vi "Dashboard Main.vi"() -> ()   [LabVIEW 2015]
uses:
  <vilib>/Utility/miscctls.llb/LVRowAndColumnTypeDef.ctl
  <vilib>/event_ctls.llb/eventvkey.ctl
  <vilib>/Rock Robotics/WPI/Dashboard/WPI_DashboardLogging Global.vi
  <vilib>/Rock Robotics/Network Tables/NT Read Numeric Array.vi
  <vilib>/Utility/config.llb/Write Key (String).vi
  <vilib>/Utility/config.llb/Write Key (I32).vi
  <vilib>/Utility/config.llb/NI_LVConfig.lvlib
panel:
  in  "TCP":refnum<k5>
  in  "Rec Mode":enum32{"Stop", "Record", "Playback"}(radio)
  in  "Vision":u16(ring) items=["Camera Off", "USB Camera SW", "USB Camera HW", "IP Camera"]
  out "Camera IP":string
  out "Image Message":string="Timeout in Camera Communications"
  in  "Dashboard Tab":T1(tab)
  in  "Select Auto":string(combo)
  out "NT Connection":bool
  in  "Camera Settings":T2={"Frame Rate"=30, "Compression"=30, "Size"=1} {"Frame Rate" scale=1.0..30.0; "Size" items=["640x480", "320x240", "160x120"]}
  out "MotorChart R":cluster{"Numeric":dbl, "Numeric":dbl}(graph)
  out "MotorChart L":T3(graph)
  out "MotorSliders R":cluster{"MotorSlide1":dbl, "MotorSlide2":dbl} {"MotorSlide2" scale=-1.0..1.0 scale format="%#_2e"; "MotorSlide1" scale=-1.0..1.0 scale format="%#_2e"}
  out "MotorSliders L":T4 {"MotorSlide4 2" scale=0.0..14.0 scale format="%#_2e"; "MotorSlide2" scale=-1.0..1.0 scale format="%#_2e"; "MotorSlide1" scale=-1.0..1.0 scale format="%#_2e"}
  out "Gyro":dbl(knob) scale=0.0..360.0
  out "JS1 Z":dbl(slide) scale=-1.0..1.0 scale format="%#_2e"
  out "JS1 Graph":cluster{"X":dbl, "Y":dbl}[](graph)
  out "JS1 Buttons":T5
  out "JS2 Z":dbl(slide) scale=-1.0..1.0 scale format="%#_2e"
  out "JS2 Graph":cluster{"X":dbl, "Y":dbl}[](graph)
  out "JS2 Buttons":T5
  out "Mode":T6(ring)=enum."Auto Disabled"
  in  "DB Camera Config":bool
  out "fps":dbl format="%#.1g"
  out "Mbps":dbl format="%#.1g"
  out "Mbps LED":bool
  in  "Auto-Mode":T7(ring)
  out "Satellite Speed":dbl(knob) scale=0.0..1.0
  out "Uranus Rotation in Degrees":dbl(knob) scale=0.0..360.0
  out "Uranus Distance":dbl
  out "Uranus Direction":bool
  out "Uranus Rate":dbl
  in  "Test Slider":dbl(slide) scale=0.0..100.0 scale format="%#_3g"
  in  "On/Off":bool caption="Solenoid"
  in  "Test Name":u16(ring) items=["Select the test to run..."]
  in  "Test Tree":string(tree)
  in  "Motor":cluster{"Value":dbl, "Enable":bool} {"Value" scale=-1.0..1.0 scale format="%#_3g"}
  out "Progress":T8 {"Test Progress" scale=0.0..100.0}
  in  "Rev/Fwd":cluster{"Forward":bool, "Reverse":bool}
  in  "Test Ring":u16(ring) items=["Monochrome", "Color"]
  out "Cmd Status":string
  in  "Execute Command":bool
  in  "Command Params":string[][](table)
  in  "Command Selection":i32(listbox)
  in  "CheckList":i32(listbox)
  out "Tree":string(tree)
  out "Camera Image":T9(plugin-control)
  out "Background":bool
  # "Left"
  # "Front"
  # "Right"
  # "Battery"
  # "This tab is a great place for autonomous settings and robot-specific values.\nPlace controls and indicators inside this tab and match name to\nDashboard Variables on robot. You can also delete this comment."
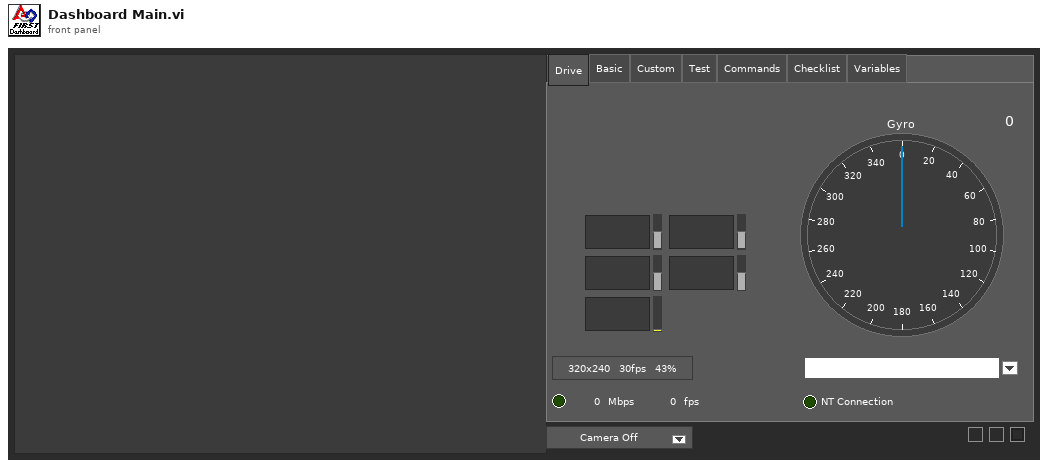
[diagram p1: front panel]
types:
  T1 = enum32{"Drive", "Basic", "Custom", "Test", "Commands", "Checklist", "Variables"}
  T2 = cluster{"Frame Rate":i32, "Compression":i32, "Size":u16}
  T3 = cluster{"Numeric":dbl, "Numeric":dbl, "Battery V":dbl}
  T4 = cluster{"MotorSlide1":dbl, "MotorSlide2":dbl, "MotorSlide4 2":dbl}
  T5 = cluster{bool, bool, bool, bool, bool, bool, bool, bool, bool, bool, bool, bool}
  T6 = enum8{"Tele-Op Disabled", "Tele-Op Enabled", "Auto Disabled", "Auto Enabled", "Test Disabled", "Test Enabled", "Disconnected", "No Code", "E-Stop"}
  T7 = enum16{"Drive-Over Stuff", "Drawbridge", "Portiwhatnot"}
  T8 = cluster{"Test Progress":u8, "Test Progress Text":string}
  T9 = typedef "IMAQ Image.ctl" = refnum<image>
  T10 = cluster{"IDs":cluster{"RPC field ID":u16, "Unique ID":u16}, "String":string}
  T11 = enum32{"Drive", "Basic", "Custom", "Test", "Checklist", "Variables"}
  T12 = typedef "Image Type" = u32
  T13 = cluster{"Camera Image":refnum<vi>, "Dashboard Tab":refnum<vi>, "Background":refnum<vi>, "Vision":refnum<vi>, "Rec Mode":refnum<vi>, "Test Slider":refnum<vi>, "On/Off ":refnum<vi>, "Test Ring":refnum<vi>, "Rev/Fwd":refnum<vi>, "Test Name":refnum<vi>, "Motor":refnum<vi>, "Progress":refnum<vi>, "CheckList":refnum<vi>, "Tree":refnum<vi>, "Test Tree":refnum<vi>, "Command Params":refnum<vi>, "Command Selection":refnum<vi>, "Execute Command":refnum<vi>, "Cmd Status":refnum<vi>}
  T14 = cluster{"Error Strings":string, "Disable Counts":cluster{u16, u16}, "Rail Faults":cluster{u16, u16, u16}, "Robot IP":string, "DB Mode":u8, "Event Info":cluster{"Name":string, "Type":u8, "Number":u16, "Replay":u8}, "Camera Addr":string}
  T15 = cluster{"Storage":cluster{"Disk Free":u64, "RAM Block":u32, "RAM free":u32}, "CPU Utilization":cluster{"CPU % ISR":sgl, "CPU % Time Crit":sgl, "CPU % Timed Str":sgl, "CPU % High":sgl, "CPU % Above":sgl, "CPU % Normal":sgl, "CPU % Low":sgl}, "CAN":cluster{"% Bus Utilization":sgl, "Bus Off Cnt":u32, "TX_FIFO Full Cnt":u32, "Receive Error Cnt":u8, "Transmit Error Cnt":u8}, "HID":cluster{"HID Outputs":u32, "Rumble Low":u16, "Rumble High":u16}[]}
  T16 = cluster{"Status bits":cluster{"Test Mode":bool, "Autonomous":bool, "Enabled":bool, "Code Start":bool, "Brownout":bool, "Reserved 2":bool, "Reserved 3":bool, "E-Stop":bool}, "Code Trace":cluster{"Disabled":bool, "TeleOp":bool, "Auto":bool, "Test":bool}, "Controller Type":enum16{"unknown", "cRIO", "roboRio"}, "Code?":enum16{"unknown", "noCode", "code"}, "Battery V":dbl}
  T17 = cluster{"Control Bits":cluster{"TestMode":bool, "Autonomous":bool, "Enabled":bool, "FMS Present":bool, bool, bool, bool, "E-Stop":bool}, "Team Station ":u8, "Countdown":sgl, "Joystick Values":cluster{"Axes":dbl[], "Buttons":bool[], "POVs":i16[]}[]}
  T18 = cluster{"Axes":dbl[], "Buttons":bool[], "POVs":i16[]}[]
  T19 = cluster{"Axes":dbl[], "Buttons":bool[], "POVs":i16[]}
  T20 = cluster{"Buttons[0]":bool, "Buttons[1]":bool, "Buttons[2]":bool, "Buttons[3]":bool, "Buttons[4]":bool, "Buttons[5]":bool, "Buttons[6]":bool, "Buttons[7]":bool, "Buttons[8]":bool, "Buttons[9]":bool, "Buttons[10]":bool, "Buttons[11]":bool}
  T21 = typedef "NI_LVConfig.lvlib/Config Data RefNum.ctl" = refnum<k1>
  T22 = cluster{"Operation":enum16{"Update", "Clear"}, "Color Box":u32}[]
  T23 = typedef "eventvkey.ctl" = enum16{"ASCII", "Enter", "Return", "Shift", "Ctrl", "Alt", "Cmd", "Opt", "Caps", "NumLock", "Clear", "Break", "Up", "Down", "Left", "Right", "Insert", "Delete", "Home", "End", "PageUp", "PageDown", "Escape", "Help", "Pause", "ScrollLock", "F1", "F2", "F3", "F4", "F5", "F6", "F7", "F8", "F9", "F10", "F11", "F12", "F13", "F14", "F15", "F16", "F17", "F18", "F19", "F20", "F21", "F22", "F23", "F24", "Play", "VolumeUp", "VolumeDown", "Mute", "Two Byte Char"}
  T24 = cluster{"Image Size":bool, "Image Type":bool, "Pixel Value":bool, "ROI Information":bool, "Zoom Factor":bool}
  T25 = enum8{"Enabled", "Disabled", "Disabled and Grayed Out"}
  T26 = cluster{"Operation":enum16{"Update", "Clear"}, "Color Box":u32}
  T27 = typedef "LVRowAndColumnTypeDef.ctl" = cluster{"Row":i32, "Column":i32}
  T28 = cluster{"Shift":bool, "Ctrl":bool, "Alt":bool, "Cmd":bool, "Opt":bool}
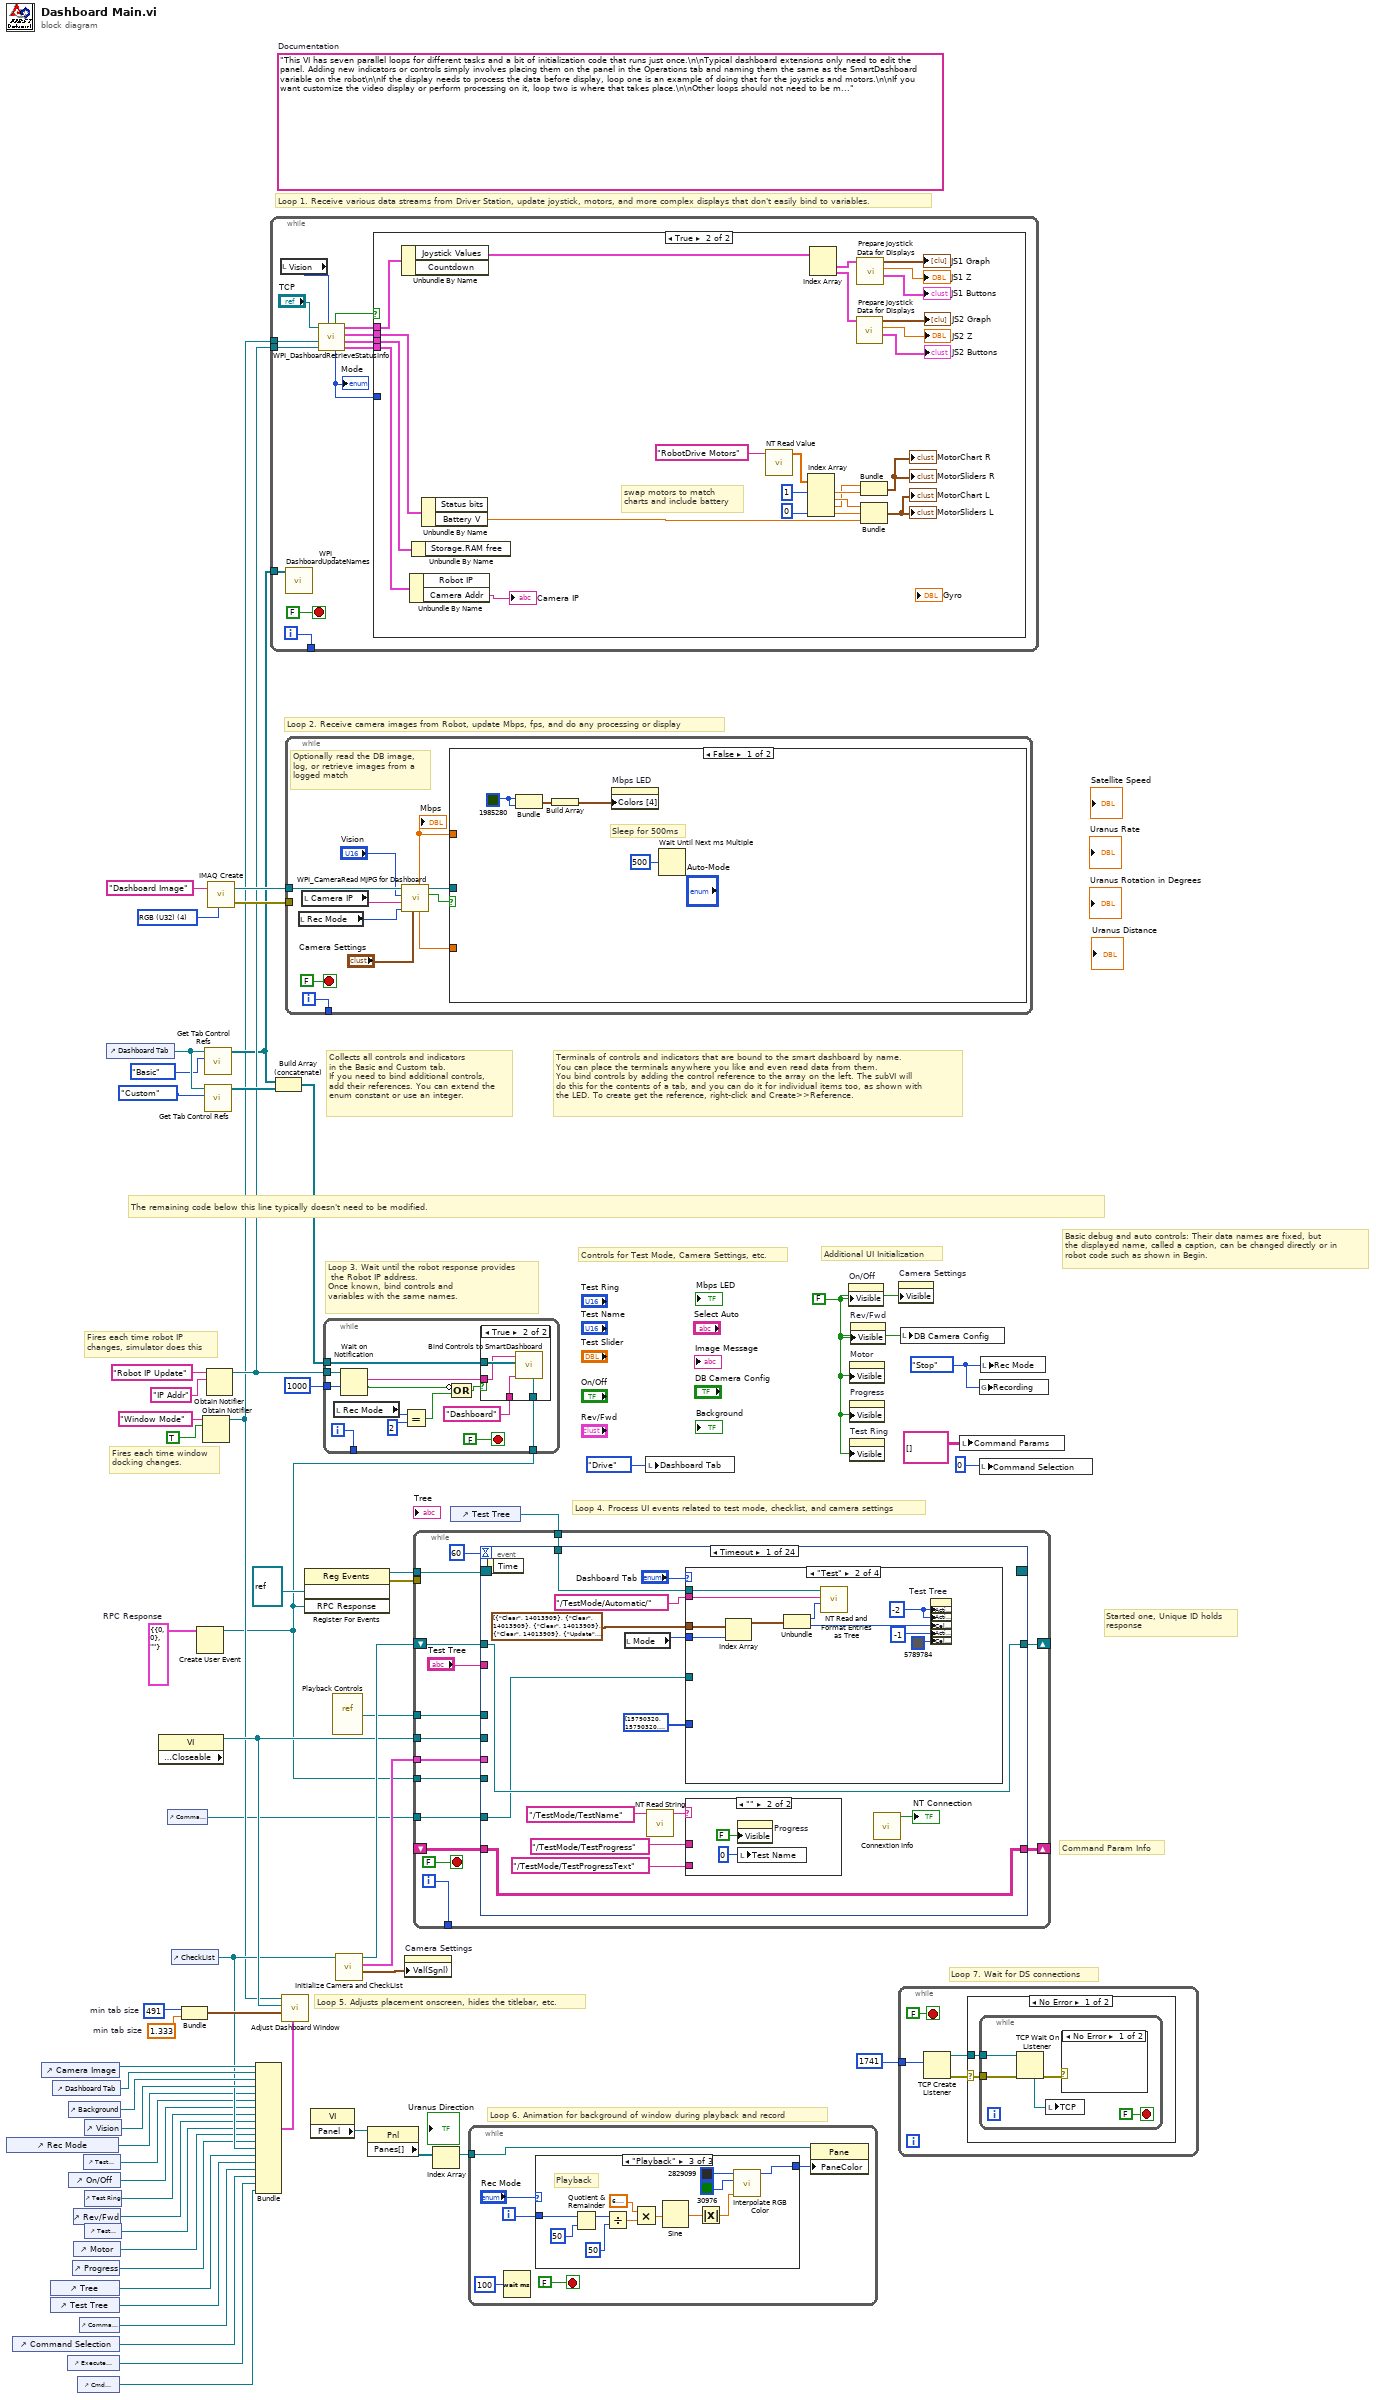
[diagram p0: block diagram]
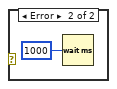
[diagram p2: hidden frame]
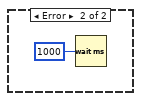
[diagram p3: hidden frame]
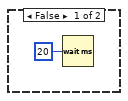
[diagram p4: hidden frame]
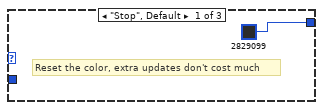
[diagram p5: hidden frame]
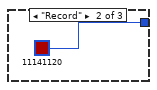
[diagram p6: hidden frame]
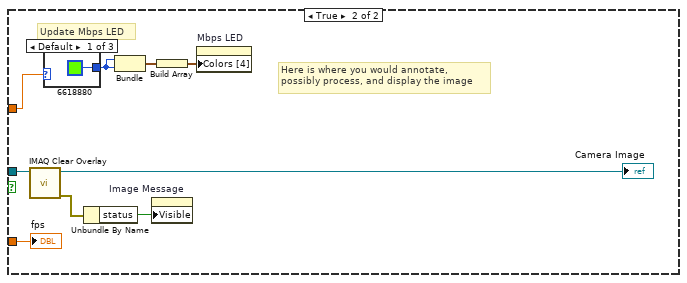
[diagram p8: hidden frame]
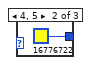
[diagram p9: hidden frame]
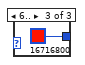
[diagram p10: hidden frame]
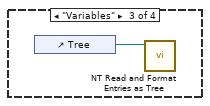
[diagram p12: hidden frame]
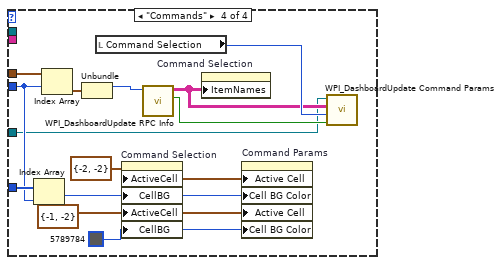
[diagram p13: hidden frame]
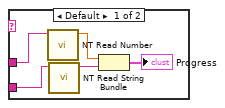
[diagram p14: hidden frame]
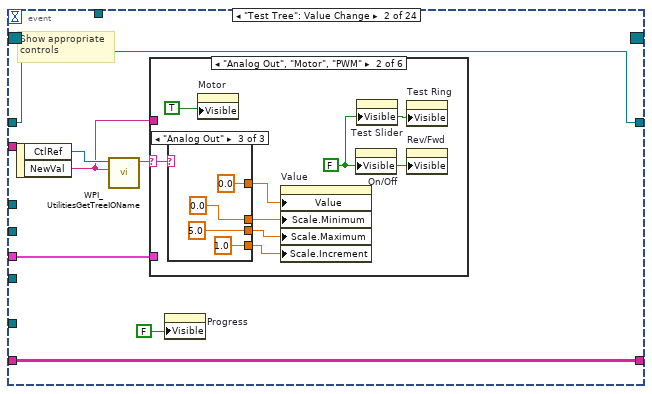
[diagram p15: hidden frame]
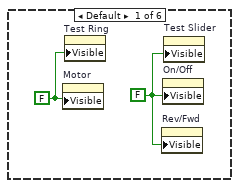
[diagram p16: hidden frame]
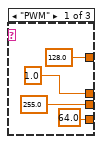
[diagram p17: hidden frame]
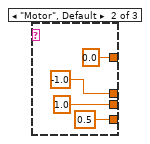
[diagram p18: hidden frame]
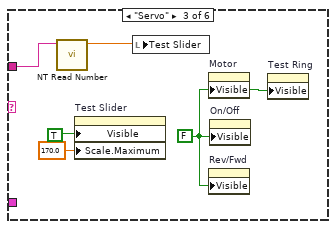
[diagram p19: hidden frame]
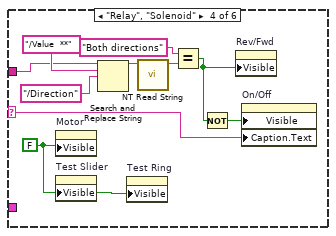
[diagram p20: hidden frame]
diagram:
  w7 = T10 {"IDs"={"RPC field ID"=0, "Unique ID"=0}, "String"=""}  # RPC Response
  w33 = 491  # min tab size
  w32 = 1.333  # min tab size
  w41 = enum32{"Stop", "Record", "Playback"}."Stop" ("Rec Mode")
  w15 = FALSE ("Visible")
  (unwired) "This VI has seven parallel loops for different tasks and a bit of initialization code that runs just once.\n\nTypical dashboard extensions only need to edit the panel. Adding new indicators or controls simply involves placing them on the panel in the Operations tab and naming them the same as the SmartDashboard variable on the robot\n\nIf the display needs to process the data before display, loop one is an example of doing that for the joysticks and motors.\n\nIf you want customize the video display or perform processing on it, loop two is where that takes place.\n\nOther loops should not need to be modified. They are pretty standard, and document the task they perform."  # Documentation
  w61 = T12 4 items=["Grayscale (U8)", "Grayscale (I16)", "Grayscale (SGL)", "Complex (CSG)", "RGB (U32)", "HSL (U32)", "RGB (U64)"] ("Image Type")
  # "Command Param Info"
  # "Started one, Unique ID holds\nresponse"
  # "Loop 7. Wait for DS connections"
  # "Basic debug and auto controls: Their data names are fixed, but\nthe displayed name, called a caption, can be changed directly or in\nrobot code such as shown in Begin."
  # "Controls for Test Mode, Camera Settings, etc."
  # "Additional UI Initialization"
  # "Loop 6. Animation for background of window during playback and record"
  # "Fires each time robot IP\nchanges, simulator does this"
  # "Fires each time window\ndocking changes."
  # "Collects all controls and indicators\nin the Basic and Custom tab.\nIf you need to bind additional controls,\nadd their references. You can extend the\nenum constant or use an integer."
  # "The remaining code below this line typically doesn't need to be modified."
  # "Loop 4. Process UI events related to test mode, checklist, and camera settings"
  # "Terminals of controls and indicators that are bound to the smart dashboard by name.\nYou can place the terminals anywhere you like and even read data from them.\nYou bind controls by adding the control reference to the array on the left. The subVI will\ndo this for the contents of a tab, and you can do it for individual items too, as shown with\nthe LED. To create get the reference, right-click and Create>>Reference."
  # "Loop 3. Wait until the robot response provides\n the Robot IP address.\nOnce known, bind controls and\nvariables with the same names."
  # "Loop 5. Adjusts placement onscreen, hides the titlebar, etc."
  # "Loop 1. Receive various data streams from Driver Station, update joystick, motors, and more complex displays that don't easily bind to variables."
  # "Loop 2. Receive camera images from Robot, update Mbps, fps, and do any processing or display"
  n1 = control-ref of="Rec Mode"() -> (w21:refnum<vi>)
  n2 = control-ref of="Command Selection"() -> (w6:refnum<vi>)
  n3 = control-ref of="Camera Image"() -> (w36:refnum<vi>)
  n4 = control-ref of="Tree"() -> (w25:refnum<vi>)
  n5 = control-ref of="Test Tree"() -> (w24:refnum<vi>)
  n6 = control-ref of="Dashboard Tab"() -> (w35:refnum<vi>)
  n7 = control-ref of="Execute Command"() -> (w8:refnum<vi>)
  n8 = control-ref of="Background"() -> (w30:refnum<vi>)
  n9 = control-ref of="On/Off"() -> (w19:refnum<vi>)
  n10 = control-ref of="Progress"() -> (w16:refnum<vi>)
  n11 = control-ref of="Rev/Fwd"() -> (w17:refnum<vi>)
  n12 = control-ref of="Motor"() -> (w22:refnum<vi>)
  n13 = control-ref of="Cmd Status"() -> (w2:refnum<vi>)
  n14 = control-ref of="Command Params"() -> (w9:refnum<vi>)
  n15 = control-ref of="Test Slider"() -> (w20:refnum<vi>)
  n16 = control-ref of="Vision"() -> (w34:refnum<vi>)
  n17 = control-ref of="Test Ring"() -> (w18:refnum<vi>)
  n18 = control-ref of="Test Name"() -> (w23:refnum<vi>)
  n19 = control-ref of="Dashboard Tab"() -> (w39:refnum<vi>)
  n20 = property class="VI" props=["Front Panel.Closeable"]() -> (reference out=w40:refnum<vi>)  [unwired: 2 in, 2 out]
  n21 = control-ref of="Command Params"() -> (w1:refnum<vi>)
  n22 = control-ref of="CheckList"() -> (w26:refnum<vi>)
  n23 = Bundle("min tab size"=w33, "min tab size"=w32) -> (w31:cluster{"min tab size":i32, "min tab size":dbl})  [unwired: 1 in]
  n24 = Create User Event(user event datatype=w7) -> (user event=w3:refnum<user-event>)  [unwired: 1 in, 1 out]
  n25 = Obtain Notifier(name (unnamed)="Window Mode", notification data type=TRUE) -> (notifier out=w12:refnum<notifier>)  [unwired: 2 in, 2 out]
  n26 = call <vilib>:"Get Tab Control Refs.vi"("Page Index"=T11."Basic" ("Dashboard Tab"), "TabControl in"=w39) -> ("ControlsOnPage"=w13:refnum<vi>[])  [unwired: 9 in]
  n27 = call <vilib>:"Get Tab Control Refs.vi"("Page Index"=T11."Custom" ("Dashboard Tab"), "TabControl in"=w39) -> ("ControlsOnPage"=w38:refnum<vi>[])  [unwired: 9 in]
  n28 = Obtain Notifier(name (unnamed)="Robot IP Update", notification data type="IP Addr" ("name (unnamed)")) -> (notifier out=w14:refnum<notifier>)  [unwired: 2 in, 2 out]
  n29 = call "IMAQ Create"("Image Name"="Dashboard Image", "Image Type"=w61) -> ("New Image"=w59:T9, "error out"=w58:errorcluster)  [unwired: 2 in, 1 out]
  n30 = Bundle("Camera Image"=w36, "Dashboard Tab"=w35, "Background"=w30, "Vision"=w34, "Rec Mode"=w21, "Test Slider"=w20, "On/Off"=w19, "Test Ring"=w18, "Rev/Fwd"=w17, "Test Name"=w23, "Motor"=w22, "Progress"=w16, "CheckList"=w26, "Tree"=w25, "Test Tree"=w24, "Command Params"=w9, "Command Selection"=w6, "Execute Command"=w8, "Cmd Status"=w2) -> (w27:T13)  [unwired: 1 in]
  n31 = while {
    tunnel: [w73] -> _
    tunnel: w14 -> [w67]
    tunnel: w13 -> [w66]
    tunnel: w12 -> [w62]
    i -> [w73]
    stop <- FALSE stop-if-true
    n32 = local read "Vision"() -> (w64:u16)
    n33 = call <vilib>:"WPI_DashboardUpdateNames.vi"("Controls on Tab"=w66) -> ()  [unwired: 11 in]
    n34 = call <vilib>:"WPI_DashboardRetrieveStatusInfo.vi"("Vision"=w64, "Binding Refnum"=w67, "Window Mode Notifier"=w62, "TCP Cnx"="TCP") -> ("Power and Errors"=w68:T14, "Robot Metrics"=w71:T15, "Status Info"=w72:T16, "Control Info"=w69:T17, "Robot Mode"=w65:T6, "Process?"=w70:bool)  [unwired: 2 in]
    "Mode" <- w65
    n35 = case shown="True" w70 {
      tunnel: w72 -> [_ w100]
      tunnel: w71 -> [_ w99]
      tunnel: w69 -> [_ w98]
      tunnel: w68 -> [_ w97]
      tunnel: w65 -> [_ _]
      frame False {
        n36 = Wait (ms)(milliseconds to wait=u32 20) -> ()  [unwired: 1 out]
      }
      frame True {
        # "swap motors to match\ncharts and include battery"
        n37 = Unbundle By Name(w98) -> ("Joystick Values"=w87:T18)  [unwired: 1 out]
        n38 = Unbundle By Name(w97) -> ("Camera Addr"=→"Camera IP":string)  [unwired: 1 out]
        n39 = Unbundle By Name(w99) -> ()  [unwired: 1 out]
        n40 = Unbundle By Name(w100) -> ("Battery V"=w88:dbl)  [unwired: 1 out]
        n41 = call-poly <vilib>:"NT Read Value.vi"("Name"="RobotDrive Motors") -> ("Numeric Array"=w76:dbl[])  [unwired: 9 in, 1 out]
        n42 = Index Array(array=w76, index #1=1, index #4=0) -> (element #1=w92:dbl, element #2=w93:dbl, element #3=w91:dbl, element #4=w96:dbl)  [unwired: 2 in]
        n43 = Index Array(array=w87) -> (element #1=w86:T19, element #2=w81:T19)  [unwired: 2 in]
        n44 = call "Prepare Joystick Data for Displays.vi"("Joystick Values"=w81) -> ("Buttons"=→"JS2 Buttons":T20, "Z Axis"=→"JS2 Z":dbl, "Cartesian Data"=→"JS2 Graph":cluster{"X axis":dbl, "X axis":dbl}[])  [unwired: 8 in]
        n45 = call "Prepare Joystick Data for Displays.vi"("Joystick Values"=w86) -> ("Buttons"=→"JS1 Buttons":T20, "Z Axis"=→"JS1 Z":dbl, "Cartesian Data"=→"JS1 Graph":cluster{"X axis":dbl, "X axis":dbl}[])  [unwired: 8 in]
        n46 = Bundle("Numeric"=w91, "Numeric"=w92) -> (→"MotorChart R" →"MotorSliders R":cluster{"Numeric":dbl, "Numeric":dbl})  [unwired: 1 in]
        n47 = Bundle("Numeric"=w93, "Numeric"=w96, "Battery V"=w88) -> (→"MotorChart L" →"MotorSliders L":T3)  [unwired: 1 in]
      }
    }
  }
  n48 = Build Array (concatenate)(w13, w38) -> (w37:refnum<vi>[])
  n49 = call "Adjust Dashboard Window.vi"("Sizing Refnums"=w27, "Size Constraints"=w31, "VI"=w40, "WIn Mode"=w12) -> ()  [unwired: 8 in]
  n50 = while {
    tunnel: w59 -> [w109]
    tunnel: w58 -> [_]
    tunnel: [w110] -> _
    i -> [w110]
    stop <- FALSE stop-if-true
    # "Optionally read the DB image,\nlog, or retrieve images from a\nlogged match"
    n51 = local read "Rec Mode"() -> (w104:enum32{"Stop", "Record", "Playback"})
    n52 = local read "Camera IP"() -> (w102:string)
    n53 = call <vilib>:"WPI_CameraRead MJPG for Dashboard.vi"("Camera Settings"="Camera Settings", "Rec Mode"=w104, "Camera IP"=w102, "Camera Mode"="Vision", "Refnum in"=w109) -> ("Active"=w107:bool, "Refnum out"=w108:T9, "FPS"=w106:dbl, "Bandwidth (Mbps)"=w101:dbl)  [unwired: 3 in]
    "Mbps" <- w101
    n54 = case shown="False" w107 {
      tunnel: w108 -> [_ w119]
      tunnel: w101 -> [_ w118]
      tunnel: w106 -> [_ w116]
      frame False {
        w112 = u32 1985280 ("Color Box")
        # "Sleep for 500ms"
        n55 = Bundle("Color Box"=w112, "Color Box"=w112) -> (w114:cluster{"Color Box":u32, "Color Box":u32})  [unwired: 1 out]
        n56 = Build Array(w114) -> (w113:cluster{"Color Box":u32, "Color Box":u32}[])
        n57 = property on="Mbps LED" class="Bool (strict)"("Colors [4]"=w113) -> ()  [unwired: 2 in, 2 out]
        n58 = Wait Until Next ms Multiple(millisecond multiple=u32 500) -> ()  [unwired: 1 out]
      }
      frame True {
        # "Here is where you would annotate,\npossibly process, and display the image"
        # "Update Mbps LED"
        n59 = call "IMAQ Clear Overlay"("Image"=w119) -> ("error out"=w123:errorcluster, "Image Out"=→"Camera Image":T9)  [unwired: 2 in, 7 out]
        n60 = case shown="Default" w118 {
          tunnel: [u32 6618880 ("Color Box") u32 16776722 ("Color Box") u32 16716800 ("Color Box")] -> w120
          frame Default {
          }
          frame 4, 5 {
          }
          frame 6.. {
          }
        }
        n61 = Unbundle By Name(w123) -> ("status"=w124:bool)
        n62 = Bundle("Color Box"=w120, "Color Box"=w120) -> (w122:cluster{"Color Box":u32, "Color Box":u32})  [unwired: 1 out]
        n63 = property on="Image Message" class="Str"("Visible"=w124) -> ()  [unwired: 2 in, 2 out]
        n64 = Build Array(w122) -> (w121:cluster{"Color Box":u32, "Color Box":u32}[])
        n65 = property on="Mbps LED" class="Bool (strict)"("Colors [4]"=w121) -> ()  [unwired: 2 in, 2 out]
        "fps" <- w116
      }
    }
  }
  n66 = register-events(refnum<vi> refnum, w3) -> (reference out=w45:refnum<event-registration>, error out=w44:errorcluster)  [unwired: 2 in]
  n67 = property class="VI"() -> ("Panel"=w48:refnum<vi>)  [unwired: 2 in, 2 out]
  n68 = while {
    tunnel: w37 -> [w140]
    tunnel: w14 -> [w138]
    tunnel: [w136] -> _
    tunnel: u32 1000 ("milliseconds to wait") -> [w135]
    tunnel: w3 -> [w128]
    i -> [w136]
    stop <- FALSE stop-if-true
    n69 = local read "Rec Mode"() -> (w131:enum32{"Stop", "Record", "Playback"})
    n70 = Wait on Notification(notifier=w138, timeout in ms (-1)=w135) -> (notification=w137:string, timed out?=w133:bool)  [unwired: 2 in, 2 out]
    n71 = Equal?(x=w131, y=u16 2 ("Rec Mode")) -> (x = y?=w132:bool)
    n72 = Compound Arithmetic op=OR(invert w133, w132) -> (w134:bool)
    n73 = case shown="True" w134 {
      tunnel: w140 -> [_ w144]
      tunnel: w137 -> [_ w143]
      tunnel: "Dashboard" -> [_ w142]
      tunnel: w128 -> [_ w141]
      frame False {
      }
      frame True {
        n74 = call <vilib>:"Bind Controls to SmartDashboard.vi"("RPC ref"=w141, "Client Name"=w142, "Bound Control Refs"=w144, "Server IP Address"=w143) -> ()  [unwired: 8 in]
      }
    }
  }
  n75 = vi-ref "Playback Controls.vi"() -> (w46:refnum<vi>)
  n76 = call "Initialize Camera and CheckList.vi"("ListBox in"=w26) -> ("Cluster"=w52:cluster{"value":i32, "value":i32, "index":i32}, "Array"=w53:cluster{string[]}[], "File Refnum"=w51:T21)  [unwired: 8 in]
  n77 = property class="Pnl"(reference=w48) -> ("Panes[]"=w49:refnum<vi>[])  [unwired: 1 in, 2 out]
  n78 = property on="Camera Settings" class="Clust (strict)"("Val(Sgnl)"=w52) -> ()  [unwired: 2 in, 2 out]
  n79 = Index Array(array=w49) -> (element=w47:refnum<vi>)  [unwired: 1 in]
  n80 = control-ref of="Test Tree"() -> (w50:refnum<vi>)
  n81 = while {
    tunnel: w53 -> [w156]
    shift-right: [w155] -> _
    shift-left: w51 -> [w154]
    tunnel: [w153] -> _
    tunnel: w50 -> [w152]
    tunnel: w46 -> [w151]
    tunnel: w45 -> [w150]
    tunnel: w44 -> [_]
    tunnel: w40 -> [w149]
    tunnel: w3 -> [w148]
    tunnel: w1 -> [w147]
    shift-right: [w146] -> _
    shift-left: _ -> [w145]
    i -> [w153]
    stop <- FALSE stop-if-true
    n82 = event shown="[0] Timeout" {
      selector: w150 -> [_ _ _ _ _ _ _ _ _ _ _ _ _ _ _ _ _ _ _ _ _ _ _ _]
      dyn-events: [_ _ _ _ _ _ _ _ _ _ _ _ _ _ _ _ _ _ w465 _ _ _ _ _] -> _
      timeout: u32 60 ("milliseconds to wait") -> [_ _ _ _ _ _ _ _ _ _ _ _ _ _ _ _ _ _ _ _ _ _ _ _]
      tunnel: w152 -> [w169 _ _ _ _ _ _ _ _ _ _ _ _ _ _ _ _ _ _ _ _ _ _ _]
      tunnel: "Test Tree" -> [_ _ _ _ _ _ _ _ _ _ _ _ _ w428 w437 w440 w445 w454 _ _ _ _ _ _]
      tunnel: w156 -> [_ w207 _ _ _ _ _ _ _ _ _ w390 w421 _ _ _ _ _ _ _ _ _ _ _]
      tunnel: [w166 w206 w310 w316 w326 w330 w336 w348 w356 w362 w375 w389 w414 w427 w435 w439 w444 w453 w467 w483 w485 w493 w504 w509] -> w155
      tunnel: w154 -> [w166 w206 w310 w316 w326 w330 w336 w348 w356 w362 w375 w388 w414 w427 w435 w439 w444 w453 w467 w483 w485 w493 w504 w509]
      tunnel: w151 -> [_ _ _ _ _ _ _ _ _ _ _ _ _ _ _ _ _ _ w468 _ w488 _ _ _]
      tunnel: w149 -> [_ _ _ _ _ _ _ _ _ _ _ _ _ _ _ _ _ _ w463 _ _ _ _ _]
      tunnel: w148 -> [_ _ _ _ _ _ _ _ _ _ _ _ _ _ _ _ _ _ w459 _ _ _ _ _]
      tunnel: w147 -> [w161 _ _ _ _ _ w334 _ _ _ _ _ _ _ _ _ _ _ _ _ _ _ _ _]
      tunnel: [w160 w205 w309 w315 w325 w331 w332 w342 w353 w361 w374 w387 w413 w426 w434 w438 w443 w452 w458 w481 w484 w489 w497 w510] -> w146
      tunnel: w145 -> [w160 w205 w309 w315 w325 w331 w332 _ _ w361 w374 w387 w413 w426 w434 w438 w443 w452 w458 w481 w484 w489 w497 w510]
      event Timeout {
        n83 = event-data() -> ()  [unwired: 1 in, 1 out]
        n84 = local read "Mode"() -> (w163:T6)
        n85 = call <vilib>:"NT Read String.vi"("Name"="/TestMode/TestName") -> ("String"=w172:string)  [unwired: 9 in, 1 out]
        n86 = case shown="\"Test\"" "Dashboard Tab" {
          tunnel: w169 -> [_ w183 _ _]
          tunnel: "/TestMode/Automatic/" ("Name Pattern") -> [_ w182 _ _]
          tunnel: T22 [{"Operation"=enum."Clear", "Color Box"=14013909}, {"Operation"=enum."Clear", "Color Box"=14013909}, {"Operation"=enum."Clear", "Color Box"=14013909}, {"Operation"=enum."Clear", "Color Box"=14013909}, {"Operation"=enum."Update", "Color Box"=14013909}, {"Operation"=enum."Update", "Color Box"=16777215}, {"Operation"=enum."Clear", "Color Box"=14013909}, {"Operation"=enum."Clear", "Color Box"=14013909}, {"Operation"=enum."Clear", "Color Box"=14013909}] -> [_ w175 _ w192]
          tunnel: w163 -> [_ w174 _ w191]
          tunnel: u32[] [15790320, 15790320, 15790320, 15790320, 16777215, 16777215, 15790320, 15790320, 15790320] -> [_ _ _ w197]
          tunnel: w161 -> [_ _ _ w185]
          frame "Custom", Default {
          }
          frame "Test" {
            w181 = -2 ("Active Item:Row Number")
            n87 = Index Array(array=w175, index=w174) -> (element=w176:T26)
            n88 = Unbundle(w176) -> ("Operation"=w177:enum16{"Update", "Clear"}, "Color Box"=w178:u32)
            n89 = call <vilib>:"NT Read and Format Entries as Tree.vi"("Operation"=w177, "Name Pattern"=w182, "Tree Refnum"=w183) -> ()  [unwired: 7 in, 2 out]
            n90 = property on="Test Tree" class="Tree (strict)"("Active Item Row Number"=w181, "ActiveColNum"=w181, "CellBG"=w178, "Active Item Row Number"=-1 ("Active Item:Row Number"), "CellBG"=u32 5789784 ("Color Box")) -> ()  [unwired: 2 in, 2 out]
          }
          frame "Variables" {
            n91 = control-ref of="Tree"() -> (w184:refnum<vi>)
            n92 = call <vilib>:"NT Read and Format Entries as Tree.vi"("Tree Refnum"=w184) -> ()  [unwired: 9 in, 2 out]
          }
          frame "Commands" {
            w193 = u32 5789784 ("Color Box")
            w194 = T27 {"Row"=-1, "Column"=-2} ("Active Cell:Active Cell")
            w196 = T27 {"Row"=-2, "Column"=-2} ("Active Cell:Active Cell")
            n93 = Index Array(array=w197, index=w191) -> (element=w195:u32)
            n94 = Index Array(array=w192, index=w191) -> (element=w190:T26)
            n95 = Unbundle(w190) -> ("Operation"=w189:enum16{"Update", "Clear"})  [unwired: 1 out]
            n96 = local read "Command Selection"() -> (w188:i32)
            n97 = property on="Command Selection" class="MCListbox (strict)"("ActiveCell"=w196, "CellBG"=w195, "ActiveCell"=w194, "CellBG"=w193) -> ()  [unwired: 2 in, 2 out]
            n98 = call <vilib>:"WPI_DashboardUpdate RPC Info.vi"("Operation"=w189) -> ("update"=w187:bool, "commands"=w186:string[][])  [unwired: 9 in]
            n99 = property on="Command Selection" class="MCListbox (strict)"("ItemNames"=w186) -> ()  [unwired: 2 in, 2 out]
            n100 = property on="Command Params" class="Tbl (strict)"("Active Cell"=w196, "Cell BG Color"=w195, "Active Cell"=w194, "Cell BG Color"=w193) -> ()  [unwired: 2 in, 2 out]
            n101 = call <vilib>:"WPI_DashboardUpdate Command Params.vi"("Update"=w187, "NewVal"=w188, "Commands"=w186, "Param Tbl"=w185) -> ()  [unwired: 7 in, 1 out]
          }
        }
        n102 = case shown="\"\"" w172 {
          tunnel: "/TestMode/TestProgress" ("Name") -> [w199 _]
          tunnel: "/TestMode/TestProgressText" ("Name") -> [w198 _]
          frame Default {
            n103 = call <vilib>:"NT Read Number.vi"("Name"=w199) -> ("Numeric"=w200:dbl)  [unwired: 9 in, 1 out]
            n104 = call <vilib>:"NT Read String.vi"("Name"=w198) -> ("String"=w201:string)  [unwired: 9 in, 1 out]
            n105 = Bundle("Numeric"=w200, "String"=w201) -> (→"Progress":cluster{"Numeric":dbl, "String":string})  [unwired: 1 in]
          }
          frame "" {
            n106 = property on="Progress" class="Clust (strict)"("Visible"=FALSE) -> ()  [unwired: 2 in, 2 out]
            n107 = local write "Test Name"(u16 0) -> ()
          }
        }
        n108 = call <vilib>:"Connextion Info.vi"() -> ("Connected"=→"NT Connection":bool)  [unwired: 10 in, 1 out]
      }
      event "Test Tree": Value Change {
        # "Show appropriate\ncontrols"
        n109 = event-data() -> ("CtlRef"=w210:refnum<vi>, "NewVal"=w208:string)  [unwired: 1 in]
        n110 = call <vilib>:"WPI_UtilitiesGetTreeIOName.vi"("NewVal"=w208, "TreeControl in"=w210) -> ("I/O Name"=w211:string)  [unwired: 9 in]
        n111 = case shown="\"Analog Out\", \"Motor\", \"PWM\"" w211 {
          selector: w211 -> [_ w218 _ w240 w249 _]
          tunnel: w208 -> [_ _ w237 w239 _ w256]
          tunnel: w207 -> [_ _ _ _ _ w255]
          frame Default {
            w213 = FALSE ("Visible")
            w212 = FALSE ("Visible")
            n112 = property on="Motor" class="Clust (strict)"("Visible"=w212) -> ()  [unwired: 2 in, 2 out]
            n113 = property on="Test Ring" class="Ring (strict)"("Visible"=w212) -> ()  [unwired: 2 in, 2 out]
            n114 = property on="Rev/Fwd" class="Clust (strict)"("Visible"=w213) -> ()  [unwired: 2 in, 2 out]
            n115 = property on="On/Off" class="Bool (strict)"("Visible"=w213) -> ()  [unwired: 2 in, 2 out]
            n116 = property on="Test Slider" class="Slide (strict)"("Visible"=w213) -> ()  [unwired: 2 in, 2 out]
          }
          frame "Analog Out", "Motor", "PWM" {
            w219 = FALSE ("Visible")
            n117 = case shown="\"Analog Out\"" w218 {
              tunnel: [1.0 ("Value") -1.0 ("Value") 0.0 ("Value")] -> w217
              tunnel: [255.0 ("Value") 1.0 ("Value") 5.0 ("Value")] -> w216
              tunnel: [128.0 ("Value") 0.0 ("Value") 0.0 ("Value")] -> w215
              tunnel: [64.0 ("Value") 0.5 ("Value") 1.0 ("Value")] -> w214
              frame "PWM" {
              }
              frame "Motor", Default {
              }
              frame "Analog Out" {
              }
            }
            n118 = property on="Motor" class="Clust (strict)"("Visible"=TRUE) -> ()  [unwired: 2 in, 2 out]
            n119 = property on="Value" class="Slide (strict)"("Value"=w215, "Scale.Minimum"=w217, "Scale.Maximum"=w216, "Scale.Increment"=w214) -> ()  [unwired: 2 in, 2 out]
            n120 = property on="On/Off" class="Bool (strict)"("Visible"=w219) -> ()  [unwired: 2 in, 2 out]
            n121 = property on="Test Slider" class="Slide (strict)"("Visible"=w219) -> ()  [unwired: 2 in, 2 out]
            n122 = property on="Test Ring" class="Ring (strict)"("Visible"=w219) -> ()  [unwired: 2 in, 2 out]
            n123 = property on="Rev/Fwd" class="Clust (strict)"("Visible"=w219) -> ()  [unwired: 2 in, 2 out]
          }
          frame "Servo" {
            w235 = FALSE ("Visible")
            n124 = call <vilib>:"NT Read Number.vi"("Name"=w237) -> ("Numeric"=w236:dbl)  [unwired: 9 in, 1 out]
            n125 = property on="Test Slider" class="Slide (strict)"("Visible"=TRUE, "Scale.Maximum"=170.0 ("Scale.Range:Maximum")) -> ()  [unwired: 2 in, 2 out]
            n126 = local write "Test Slider"(w236) -> ()
            n127 = property on="Motor" class="Clust (strict)"("Visible"=w235) -> ()  [unwired: 2 in, 2 out]
            n128 = property on="Rev/Fwd" class="Clust (strict)"("Visible"=w235) -> ()  [unwired: 2 in, 2 out]
            n129 = property on="On/Off" class="Bool (strict)"("Visible"=w235) -> ()  [unwired: 2 in, 2 out]
            n130 = property on="Test Ring" class="Ring (strict)"("Visible"=w235) -> ()  [unwired: 2 in, 2 out]
          }
          frame "Relay", "Solenoid" {
            w238 = FALSE ("Visible")
            n131 = property on="Motor" class="Clust (strict)"("Visible"=w238) -> ()  [unwired: 2 in, 2 out]
            n132 = property on="Test Slider" class="Slide (strict)"("Visible"=w238) -> ()  [unwired: 2 in, 2 out]
            n133 = Search and Replace String(input string=w239, search string="/Value  **", replace string="/Direction") -> (result string=w245:string)  [unwired: 5 in, 3 out]
            n134 = property on="Test Ring" class="Ring (strict)"("Visible"=w238) -> ()  [unwired: 2 in, 2 out]
            n135 = call <vilib>:"NT Read String.vi"("Name"=w245) -> ("String"=w243:string)  [unwired: 9 in, 1 out]
            n136 = Equal?(x="Both directions", y=w243) -> (x = y?=w241:bool)
            n137 = Not(x=w241) -> (.not. x?=w242:bool)
            n138 = property on="Rev/Fwd" class="Clust (strict)"("Visible"=w241) -> ()  [unwired: 2 in, 2 out]
            n139 = property on="On/Off" class="Bool (strict)"("Visible"=w242, "Caption.Text"=w240) -> ()  [unwired: 2 in, 2 out]
          }
          frame "Compressor", "Digital Out" {
            w248 = FALSE ("Visible")
            # "Get direction and finish"
            n140 = property on="Motor" class="Clust (strict)"("Visible"=w248) -> ()  [unwired: 2 in, 2 out]
            n141 = property on="Test Slider" class="Slide (strict)"("Visible"=w248) -> ()  [unwired: 2 in, 2 out]
            n142 = property on="Test Ring" class="Ring (strict)"("Visible"=w248) -> ()  [unwired: 2 in, 2 out]
            n143 = property on="On/Off" class="Bool (strict)"("Visible"=TRUE, "Caption.Text"=w249) -> ()  [unwired: 2 in, 2 out]
            n144 = property on="Rev/Fwd" class="Clust (strict)"("Visible"=FALSE) -> ()  [unwired: 2 in, 2 out]
          }
          frame "Camera" {
            n145 = call <vilib>:"Get Last Path Segment.vi"("String in"=w256) -> ("String out"=w257:string)  [unwired: 10 in]
            n146 = property on="On/Off" class="Bool (strict)"("Visible"=FALSE) -> ()  [unwired: 2 in, 2 out]
            n147 = property on="Motor" class="Clust (strict)"("Visible"=FALSE) -> ()  [unwired: 2 in, 2 out]
            n148 = property on="Rev/Fwd" class="Clust (strict)"("Visible"=FALSE) -> ()  [unwired: 2 in, 2 out]
            n149 = case shown="\"White Balance  **\"" w257 {
              tunnel: w256 -> [w263 w272 w281 w290 w299 _ w305]
              tunnel: w255 -> [w261 w269 w278 w287 w296 _ _]
              frame "Size  **" {
                n150 = Index Array(array=w261) -> (element=w260:cluster{string[]})  [unwired: 1 in]
                n151 = call <vilib>:"NT Read String.vi"("Name"=w263) -> ("String"=w262:string)  [unwired: 9 in, 1 out]
                n152 = Unbundle(w260) -> (w258:string[])
                n153 = Match First String(2:w258, 3:w262) -> (0:w259:i32)  [unwired: 1 out]
                n154 = property on="Test Ring" class="Ring (strict)"("Value"=w259, "Strings []"=w258) -> ()  [unwired: 2 in, 2 out]
                n155 = property on="Test Ring" class="Ring (strict)"("Visible"=TRUE) -> ()  [unwired: 2 in, 2 out]
                n156 = property on="Test Slider" class="Slide (strict)"("Visible"=FALSE) -> ()  [unwired: 2 in, 2 out]
              }
              frame "White Balance  **" {
                n157 = Index Array(array=w269, index=1) -> (element=w270:cluster{string[]})
                n158 = call <vilib>:"NT Read String.vi"("Name"=w272) -> ("String"=w271:string)  [unwired: 9 in, 1 out]
                n159 = Unbundle(w270) -> (w267:string[])
                n160 = Match First String(2:w267, 3:w271) -> (0:w266:i32)  [unwired: 1 out]
                n161 = property on="Test Ring" class="Ring (strict)"("Value"=w266, "Strings []"=w267) -> ()  [unwired: 2 in, 2 out]
                n162 = property on="Test Ring" class="Ring (strict)"("Visible"=TRUE) -> ()  [unwired: 2 in, 2 out]
                n163 = property on="Test Slider" class="Slide (strict)"("Visible"=FALSE) -> ()  [unwired: 2 in, 2 out]
              }
              frame "Exposure  **" {
                n164 = Index Array(array=w278, index=2) -> (element=w279:cluster{string[]})
                n165 = call <vilib>:"NT Read String.vi"("Name"=w281) -> ("String"=w280:string)  [unwired: 9 in, 1 out]
                n166 = Unbundle(w279) -> (w275:string[])
                n167 = Match First String(2:w275, 3:w280) -> (0:w276:i32)  [unwired: 1 out]
                n168 = property on="Test Ring" class="Ring (strict)"("Value"=w276, "Strings []"=w275) -> ()  [unwired: 2 in, 2 out]
                n169 = property on="Test Ring" class="Ring (strict)"("Visible"=TRUE) -> ()  [unwired: 2 in, 2 out]
                n170 = property on="Test Slider" class="Slide (strict)"("Visible"=FALSE) -> ()  [unwired: 2 in, 2 out]
              }
              frame "Exposure Priority  **" {
                n171 = Index Array(array=w287, index=3) -> (element=w288:cluster{string[]})
                n172 = call <vilib>:"NT Read String.vi"("Name"=w290) -> ("String"=w289:string)  [unwired: 9 in, 1 out]
                n173 = Unbundle(w288) -> (w284:string[])
                n174 = Match First String(2:w284, 3:w289) -> (0:w285:i32)  [unwired: 1 out]
                n175 = property on="Test Ring" class="Ring (strict)"("Value"=w285, "Strings []"=w284) -> ()  [unwired: 2 in, 2 out]
                n176 = property on="Test Ring" class="Ring (strict)"("Visible"=TRUE) -> ()  [unwired: 2 in, 2 out]
                n177 = property on="Test Slider" class="Slide (strict)"("Visible"=FALSE) -> ()  [unwired: 2 in, 2 out]
              }
              frame "Color Enable  **" {
                n178 = Index Array(array=w296, index=4) -> (element=w297:cluster{string[]})
                n179 = call <vilib>:"NT Read String.vi"("Name"=w299) -> ("String"=w298:string)  [unwired: 9 in, 1 out]
                n180 = Unbundle(w297) -> (w293:string[])
                n181 = Match First String(2:w293, 3:w298) -> (0:w294:i32)  [unwired: 1 out]
                n182 = property on="Test Ring" class="Ring (strict)"("Value"=w294, "Strings []"=w293) -> ()  [unwired: 2 in, 2 out]
                n183 = property on="Test Ring" class="Ring (strict)"("Visible"=TRUE) -> ()  [unwired: 2 in, 2 out]
                n184 = property on="Test Slider" class="Slide (strict)"("Visible"=FALSE) -> ()  [unwired: 2 in, 2 out]
              }
              frame Default {
                n185 = property on="Test Ring" class="Ring (strict)"("Visible"=FALSE) -> ()  [unwired: 2 in, 2 out]
                n186 = property on="Test Slider" class="Slide (strict)"("Visible"=FALSE) -> ()  [unwired: 2 in, 2 out]
              }
              frame "Brightness  **", "Color Level  **", "Compression  **", "FPS  **", "Sharpness  **" {
                n187 = call <vilib>:"NT Read Number.vi"("Name"=w305) -> ("Numeric"=w304:dbl)  [unwired: 9 in, 1 out]
                n188 = local write "Test Slider"(w304) -> ()
                n189 = property on="Test Slider" class="Slide (strict)"("Visible"=TRUE, "Scale.Maximum"=100.0 ("Scale.Range:Maximum")) -> ()  [unwired: 2 in, 2 out]
                n190 = property on="Test Ring" class="Ring (strict)"("Visible"=FALSE) -> ()  [unwired: 2 in, 2 out]
              }
            }
          }
        }
        n191 = property on="Progress" class="Clust (strict)"("Visible"=FALSE) -> ()  [unwired: 2 in, 2 out]
      }
      event "Test Name": Mouse Enter {
        # "Populate the ring with the list of tests"
        n192 = event-data() -> ()  [unwired: 1 in, 1 out]
        n193 = call <vilib>:"NT Read String Array.vi"("Name"="/TestMode/TestList") -> ("String Array"=w314:string[])  [unwired: 9 in, 1 out]
        n194 = Build Array (concatenate)("Select the test to run...", w314) -> (w313:string[])
        n195 = property on="Test Name" class="Ring (strict)"("Strings []"=w313) -> ()  [unwired: 2 in, 2 out]
      }
      event "Test Name": Value Change {
        w317 = FALSE ("Visible")
        # "Tell the robot the test name to run"
        n196 = event-data() -> ("NewVal"=w321:u16)  [unwired: 1 in]
        n197 = property on="Test Name" class="Ring (strict)"() -> ("Strings []"=w322:string[])  [unwired: 2 in, 2 out]
        n198 = local write "Progress"(T8 {"Test Progress"=0, "Test Progress Text"=""} ("Progress")) -> ()
        n199 = Index Array(array=w322, index=w321) -> (element=w320:string)
        n200 = call <vilib>:"NT Write String.vi"("String"=w320, "Name"="/TestMode/TestName") -> ()  [unwired: 9 in, 1 out]
        n201 = property on="Progress" class="Clust (strict)"("Visible"=TRUE) -> ()  [unwired: 2 in, 2 out]
        n202 = property on="Motor" class="Clust (strict)"("Visible"=w317) -> ()  [unwired: 2 in, 2 out]
        n203 = property on="Test Slider" class="Slide (strict)"("Visible"=w317) -> ()  [unwired: 2 in, 2 out]
        n204 = property on="On/Off" class="Bool (strict)"("Visible"=w317) -> ()  [unwired: 2 in, 2 out]
        n205 = property on="Rev/Fwd" class="Clust (strict)"("Visible"=w317) -> ()  [unwired: 2 in, 2 out]
        n206 = property on="Test Ring" class="Ring (strict)"("Visible"=w317) -> ()  [unwired: 2 in, 2 out]
      }
      event "Select Auto": Mouse Enter {
        # "Populate the combo box with the list of autonomous options"
        n207 = event-data() -> ()  [unwired: 1 in, 1 out]
        n208 = call <vilib>:"NT Read String Array.vi"("Name"="Auto List") -> ("String Array"=w324:string[])  [unwired: 9 in, 1 out]
        n209 = property on="Select Auto" class="CmbBox"("Strings[]"=w324) -> ()  [unwired: 2 in, 2 out]
      }
      event "Select Auto": Value Change {
        # "User modified the Auto Selection. Write to NT variable so robot knows."
        n210 = event-data() -> ("NewVal"=w328:string)  [unwired: 1 in]
        n211 = call <vilib>:"NT Write String.vi"("String"=w328, "Name"="Auto Selector") -> ()  [unwired: 9 in, 1 out]
      }
      event "Command Selection": Value Change {
        # "Get the params and show in table"
        n212 = event-data() -> ("NewVal"=w335:i32)  [unwired: 1 in]
        n213 = property on="Command Selection" class="MCListbox (strict)"() -> ("ItemNames"=w333:string[][])  [unwired: 2 in, 2 out]
        n214 = call <vilib>:"WPI_DashboardUpdate Command Params.vi"("NewVal"=w335, "Commands"=w333, "Param Tbl"=w334) -> ()  [unwired: 8 in, 1 out]
      }
      event "Execute Command": Value Change {
        # "Started one, Unique ID holds\nresponse"
        n215 = event-data() -> ()  [unwired: 1 in, 1 out]
        n216 = property on="Command Selection" class="MCListbox (strict)"() -> ("ItemNames"=w347:string[][])  [unwired: 2 in, 2 out]
        n217 = Index Array(array=w347, index (row)="Command Selection", index (col)=0) -> (element=w345:string)
        n218 = call <vilib>:"Invoke Commands.vi"("Command Params"="Command Params", "Function Name"=w345) -> ("Params"=w341:u8, "Started"=w340:bool)  [unwired: 7 in, 1 out]
        n219 = Array Subset(array="Command Params", length (row)=w341) -> (w342:string[][])  [unwired: 3 in]
        n220 = Select(t="Executing" ("Cmd Status"), s=w340, f="" ("Cmd Status")) -> (s? t:f=→"Cmd Status":string)
      }
      event "Command Selection": Double Click {
        n221 = event-data() -> ("Row"=w357:i32)  [unwired: 1 in]
        n222 = property on="Command Selection" class="MCListbox (strict)"() -> ("ItemNames"=w360:string[][])  [unwired: 2 in, 2 out]
        n223 = local read "Command Params"() -> (w355:string[][])
        n224 = Index Array(array=w360, index (row)=w357, index (col)=0) -> (element=w358:string)
        n225 = call <vilib>:"Invoke Commands.vi"("Command Params"=w355, "Function Name"=w358) -> ("Params"=w354:u8, "Started"=w349:bool)  [unwired: 7 in, 1 out]
        n226 = Array Subset(array=w355, length (row)=w354) -> (w353:string[][])  [unwired: 3 in]
        n227 = Select(t="Executing" ("Cmd Status"), s=w349, f="" ("Cmd Status")) -> (s? t:f=w350:string)
        n228 = local write "Cmd Status"(w350) -> ()
      }
      event "CheckList": Double Click {
        # "Shift clears all"
        # "Update symbols on the listbox"
        n229 = event-data() -> ("PlatMods.Shift"=w363:bool, "Row"=w365:i32)  [unwired: 1 in]
        n230 = case shown="True" w363 {
          tunnel: w365 -> [w369 _]
          tunnel: 1 -> [w368 _]
          frame False {
            n231 = property on="CheckList" class="LstBox (strict)"() -> ("Item Symbols"=w367:i32[])  [unwired: 2 in, 2 out]
            n232 = Replace Array Subset(array=w367, new element=w368, index=w369) -> (w366:i32[])
            n233 = property on="CheckList" class="LstBox (strict)"("Item Symbols"=w366) -> ()  [unwired: 2 in, 2 out]
          }
          frame True {
            w370 = 0 ("Top Row")
            n234 = property on="CheckList" class="LstBox (strict)"() -> ("Number of Rows"=w372:u32)  [unwired: 2 in, 2 out]
            n235 = Initialize Array(0, w372) -> (w371:i32[])
            n236 = property on="CheckList" class="LstBox (strict)"("Top Row"=w370, "Value"=w370, "Item Symbols"=w371) -> ()  [unwired: 2 in, 2 out]
          }
        }
      }
      event "CheckList": Key Down {
        # "Update symbols on the listbox\nLeft and right keys check and uncheck"
        n237 = event-data() -> ("VKey"=w377:T23)  [unwired: 1 in]
        n238 = case shown="\"Left\", \"Right\"" w377 {
          selector: w377 -> [w382 _]
          tunnel: eventvkey."Left" ("VKey") -> [w380 _]
          frame "Left", "Right" {
            n239 = Equal?(x=w380, y=w382) -> (x = y?=w381:bool)
            n240 = Select(t=0, s=w381, f=1) -> (s? t:f=w383:i32)
            n241 = property on="CheckList" class="LstBox (strict)"() -> ("Item Symbols"=w386:i32[])  [unwired: 2 in, 2 out]
            n242 = Replace Array Subset(array=w386, new element=w383, index="CheckList") -> (w385:i32[])
            n243 = property on="CheckList" class="LstBox (strict)"("Item Symbols"=w385) -> ()  [unwired: 2 in, 2 out]
          }
          frame Default {
          }
        }
      }
      event "DB Camera Config": Value Change {
        # "Show or hide the cluster of controls, store in ini file"
        n244 = event-data() -> ("NewVal"=w391:bool)  [unwired: 1 in]
        n245 = case shown="False" w391 {
          tunnel: w390 -> [w400 _]
          tunnel: [w393 w411] -> w389
          tunnel: w388 -> [w392 w411]
          frame False {
            w407 = "Camera"
            w410 = FALSE ("Visible")
            n246 = local read "Camera Settings"() -> (w399:T2)
            n247 = Index Array(array=w400) -> (element=w403:cluster{string[]})  [unwired: 1 in]
            n248 = Unbundle(w399) -> ("Frame Rate"=w398:i32, "Compression"=w397:i32, "Size"=w401:u16)
            n249 = Unbundle(w403) -> (w402:string[])
            n250 = Index Array(array=w402, index=w401) -> (element=w396:string)
            n251 = call-poly <vilib>:"Write Key.vi"("section"=w407, "value"=w396, "key"="Size", "refnum"=w392) -> ("refnum out"=w409:T21)  [unwired: 2 in, 5 out]
            n252 = call-poly <vilib>:"Write Key.vi"("section"=w407, "value"=w398, "key"="FrameRate", "refnum"=w409) -> ("refnum out"=w408:T21)  [unwired: 1 in, 6 out]
            n253 = property on="Camera Settings" class="Clust (strict)"("Visible"=w410) -> ()  [unwired: 2 in, 2 out]
            n254 = local write "DB Camera Config"(w410) -> ()
            n255 = call-poly <vilib>:"Write Key.vi"("section"=w407, "value"=w397, "key"="Compression", "refnum"=w408) -> ("refnum out"=w394:T21)  [unwired: 1 in, 6 out]
            n256 = call <vilib>:"Close Config Data.vi"("refnum"=w394) -> ("file path"=w395:path)  [unwired: 2 in, 8 out]
            n257 = call <vilib>:"Open Config Data.vi"("configuration file path"=w395) -> ("refnum"=w393:T21)  [unwired: 8 in, 2 out]
          }
          frame True {
            n258 = property on="Camera Settings" class="Clust (strict)"("Visible"=TRUE) -> ()  [unwired: 2 in, 2 out]
          }
        }
      }
      event "Camera Settings": Value Change {
        # "Update summary string when any elements of DB camera change"
        n259 = event-data() -> ("NewVal"=w425:T2)  [unwired: 1 in]
        n260 = Index Array(array=w421) -> (element=w420:cluster{string[]})  [unwired: 1 in]
        n261 = Unbundle(w425) -> ("Frame Rate"=w416:i32, "Compression"=w415:i32, "Size"=w418:u16)
        n262 = Unbundle(w420) -> (w419:string[])
        n263 = Index Array(array=w419, index=w418) -> (element=w417:string)
        n264 = Format Into String(format string="%s   %dfps   %d%%", w417, w416, w415) -> (resulting string=w422:string)  [unwired: 2 in, 1 out]
        n265 = Build Array(w422) -> (w423:string[])
        n266 = property on="DB Camera Config" class="Bool (strict)"("Strings [4]"=w423) -> ()  [unwired: 2 in, 2 out]
      }
      event "Motor.Enable": Value Change {
        # "When the test mode otor enable helper is set, update that\ntree row item's value"
        n267 = event-data() -> ("NewVal"=w432:bool)  [unwired: 1 in]
        n268 = Unbundle("Motor") -> ("Value"=w431:dbl)  [unwired: 1 out]
        n269 = Select(t=w431, s=w432, f=0.0) -> (s? t:f=w429:dbl)
        n270 = call <vilib>:"NT Write Number.vi"("Numeric"=w429, "Name"=w428) -> ()  [unwired: 9 in, 1 out]
      }
      event "Test Slider": Value Change {
        # "When the test mode slider helper is set, update that\ntree row item's value"
        n271 = event-data() -> ("NewVal"=w436:dbl)  [unwired: 1 in]
        n272 = call <vilib>:"NT Write Number.vi"("Numeric"=w436, "Name"=w437) -> ()  [unwired: 9 in, 1 out]
      }
      event "On/Off": Value Change {
        # "When the test mode on/off helper value is set, update that\ntree row item's value"
        n273 = event-data() -> ("NewVal"=w442:bool)  [unwired: 1 in]
        n274 = Boolean To (0,1)(Boolean=w442) -> (0, 1=w441:i16)
        n275 = call <vilib>:"NT Write Number.vi"("Numeric"=w441, "Name"=w440) -> ()  [unwired: 9 in, 1 out]
      }
      event "Rev/Fwd": Value Change {
        # "When the test mode helper value for relays is set, update that\ntree row item's value"
        n276 = event-data() -> ("NewVal.Forward"=w451:bool, "NewVal.Reverse"=w450:bool)  [unwired: 1 in]
        n277 = Boolean To (0,1)(Boolean=w451) -> (0, 1=w447:i16)
        n278 = Boolean To (0,1)(Boolean=w450) -> (0, 1=w449:i16)
        n279 = Negate(x=w449) -> (-x=w448:i16)
        n280 = Add(x=w447, y=w448) -> (x+y=w446:i16)
        n281 = call <vilib>:"NT Write Number.vi"("Numeric"=w446, "Name"=w445) -> ()  [unwired: 9 in, 1 out]
      }
      event "Test Ring": Value Change {
        # "When a test mode helper value is selected from the ring,\nset the tree item's variable to the string value"
        n282 = event-data() -> ("NewVal"=w456:u16)  [unwired: 1 in]
        n283 = property on="Test Ring" class="Ring (strict)"() -> ("Strings []"=w457:string[])  [unwired: 2 in, 2 out]
        n284 = Index Array(array=w457, index=w456) -> (element=w455:string)
        n285 = call <vilib>:"NT Write String.vi"("String"=w455, "Name"=w454) -> ()  [unwired: 9 in, 1 out]
      }
      event "Rec Mode": Value Change {
        # "Update globals for recording mode and path to read log from.\nClear when logging and let NetworkTables set path for vision to\nuse."
        n286 = event-data() -> ("NewVal"=w469:enum32{"Stop", "Record", "Playback"})  [unwired: 1 in]
        n287 = global write "WPI_DashboardLogging Global.vi" "Logging Filename"(path "") -> ()
        n288 = global write "WPI_DashboardLogging Global.vi" "Recording"(w469) -> ()
        n289 = case shown="\"Playback\"" w469 {
          tunnel: w468 -> [_ w471 w480]
          tunnel: [_ _ w479] -> w465
          tunnel: [_ _ w478] -> _
          tunnel: w463 -> [_ _ w476]
          tunnel: cluster{i32, i32} {-250, 170} -> [_ _ w475]
          tunnel: [_ _ T24 {"Image Size"=TRUE, "Image Type"=TRUE, "Pixel Value"=TRUE, "ROI Information"=TRUE, "Zoom Factor"=FALSE} ("Image Information Shown:All Elements")] -> w461
          tunnel: [_ _ TRUE ("Zoom Factor")] -> w460
          tunnel: w459 -> [_ _ w472]
          frame Default {
          }
          frame "Stop", "Record" {
            # "Place Window too"
            n290 = invoke class="VI" method="FP.Close"(reference=w471) -> (reference out=w470:refnum<vi>)  [unwired: 2 in, 2 out]
            n291 = invoke class="VI" method="Abort VI"(reference=w470) -> ()  [unwired: 2 in, 3 out]
          }
          frame "Playback" {
            n292 = call "Open Playback Panel.vi"("Offset"=w475, "DB VI Ref"=w476, "Playback in"=w480) -> ("Playback out"=w477:refnum<vi>)  [unwired: 8 in]
            n293 = register-events(w477, w472) -> (reference out=w479:refnum<event-registration>, error out=w478:errorcluster)  [unwired: 2 in]
          }
        }
        n294 = property on="Camera Image" class="ImageControl"("Image Information Shown"=w461, "Image Information Visible"=w460) -> ()  [unwired: 2 in, 2 out]
        n295 = call <vilib>:"WPI_DashboardNT Log FieldName Cache.vi"("Operation"=enum16{"Lookup/Add", "Index", "Clear"}."Clear") -> ()  [unwired: 8 in, 3 out]
      }
      event Panel Close {
        w482 = enum32{"Stop", "Record", "Playback"}."Stop" ("Rec Mode")
        # "Playback window has been closed, abort"
        n296 = event-data() -> ()  [unwired: 1 in, 4 out]
        n297 = local write "Rec Mode"(w482) -> ()
        n298 = global write "WPI_DashboardLogging Global.vi" "Recording"(w482) -> ()
      }
      event Panel Close {
        # "Abort playback window and ourself"
        n299 = event-data() -> ()  [unwired: 1 in, 4 out]
        n300 = invoke class="VI" method="FP.Close"(reference=w488) -> (reference out=w487:refnum<vi>)  [unwired: 2 in, 2 out]
        n301 = invoke class="VI" method="Abort VI"(reference=w487) -> (error out=w486:errorcluster)  [unwired: 2 in, 2 out]
        n302 = invoke class="VI" method="Abort VI"(error in=w486) -> ()  [unwired: 2 in, 3 out]
      }
      event User Event {
        n303 = event-data() -> ("IDs"=w496:cluster{"RPC field ID":u16, "Unique ID":u16}, "String"=w495:string)  [unwired: 1 in]
        n304 = Bundle("IDs"=w496, "String"=w495) -> (w494:T10)  [unwired: 1 in]
        n305 = call <vilib>:"Retrieve RPC Response.vi"("RPC Response"=w494) -> ("Output"=w491:string[][])  [unwired: 10 in]
        n306 = Build Array (concatenate)(w489, w491) -> (w490:string[][])
        n307 = local write "Command Params"(w490) -> ()
        n308 = local write "Cmd Status"("" ("Cmd Status")) -> ()
      }
      event "Vision": Value Change {
        # "Enable/Disable Compression slider.\nHW USB is hard-coded into the camera"
        n309 = event-data() -> ("NewVal"=w503:u16)  [unwired: 1 in]
        n310 = Equal?(x=w503, y=u32 2 ("milliseconds to wait")) -> (x = y?=w501:bool)
        n311 = Select(t=T25."Disabled and Grayed Out" ("Disabled"), s=w501, f=T25."Enabled" ("Disabled")) -> (s? t:f=w498:T25)
        n312 = property on="Compression" class="Slide (strict)"("DisabledEnum"=w498) -> ()  [unwired: 2 in, 2 out]
      }
      event "Tree": Double Click {
        n313 = event-data() -> ("PlatMods"=w508:T28, "Tag"=w507:string)  [unwired: 1 in]
        n314 = Unbundle(w508) -> ("Shift"=w506:bool)  [unwired: 4 out]
        n315 = Not(x=w506) -> (.not. x?=w505:bool)
        n316 = call <vilib>:"NT Update Persistence.vi"("Persistence"=w505, "Name"=w507) -> ()  [unwired: 9 in, 1 out]
      }
    }
  }
  n317 = while {
    tunnel: w47 -> [w512]
    i -> [w515]
    stop <- FALSE stop-if-true
    n318 = Wait (ms)(milliseconds to wait=u32 100) -> ()  [unwired: 1 out]
    n319 = case shown="\"Playback\"" "Rec Mode" {
      tunnel: w515 -> [_ _ w530]
      tunnel: [u32 2829099 ("Base Color") u32 11141120 ("Target Color") w519] -> w511
      frame "Stop", Default {
        # "Reset the color, extra updates don't cost much"
      }
      frame "Record" {
      }
      frame "Playback" {
        # "Playback"
        n320 = Quotient & Remainder(x=w530, y=u32 50 ("milliseconds to wait")) -> (x-y*floor(x/y)=w526:u32)  [unwired: 1 out]
        n321 = Divide(x=w526, y=u32 50 ("milliseconds to wait")) -> (x/y=w523:dbl)
        n322 = Multiply(x=6.283185307179586, y=w523) -> (x*y=w528:dbl)
        n323 = Sine(x=w528) -> (sin(x)=w527:dbl)
        n324 = Absolute Value(x=w527) -> (abs(x)=w520:dbl)
        n325 = call "Interpolate RGB Color.vi"("Proportion"=w520, "Target Color"=u32 30976, "Base Color"=u32 2829099) -> ("Result Color"=w519:u32)  [unwired: 8 in]
      }
    }
    n326 = property class="Pane"(reference=w512, "PaneColor"=w511) -> ()  [unwired: 1 in, 2 out]
  }
  n327 = local write "Dashboard Tab"(T1."Drive" ("Dashboard Tab")) -> ()
  n328 = property on="On/Off" class="Bool (strict)"("Visible"=w15) -> ()  [unwired: 2 in, 2 out]
  n329 = property on="Motor" class="Clust (strict)"("Visible"=w15) -> ()  [unwired: 2 in, 2 out]
  n330 = property on="Progress" class="Clust (strict)"("Visible"=w15) -> ()  [unwired: 2 in, 2 out]
  n331 = property on="Test Ring" class="Ring (strict)"("Visible"=w15) -> ()  [unwired: 2 in, 2 out]
  n332 = property on="Rev/Fwd" class="Clust (strict)"("Visible"=w15) -> ()  [unwired: 2 in, 2 out]
  n333 = property on="Camera Settings" class="Clust (strict)"("Visible"=w15) -> ()  [unwired: 2 in, 2 out]
  n334 = while {
    tunnel: u16 1741 ("timeout ms (25000)") -> [w532]
    stop <- FALSE stop-if-true
    n335 = TCP Create Listener(10:w532) -> (0:w531:errorcluster, 3:w533:refnum<k5>)  [unwired: 4 in, 1 out]
    n336 = case shown="No Error" w531 {
      selector: w531 -> [w535 _]
      tunnel: w533 -> [w536 _]
      frame No Error {
        n337 = while {
          tunnel: w536 -> [w539]
          tunnel: w535 -> [w538]
          stop <- FALSE stop-if-true
          n338 = TCP Wait On Listener(8:w538, 11:w539) -> (0:w540:errorcluster, 4:w541:refnum<k5>)  [unwired: 2 in, 3 out]
          n339 = local write "TCP"(w541) -> ()
          n340 = case shown="No Error" w540 {
            frame No Error {
            }
            frame Error {
              n341 = Wait (ms)(milliseconds to wait=u32 1000) -> ()  [unwired: 1 out]
            }
          }
        }
      }
      frame Error {
        n342 = Wait (ms)(milliseconds to wait=u32 1000) -> ()  [unwired: 1 out]
      }
    }
  }
  n343 = local write "DB Camera Config"(w15) -> ()
  n344 = local write "Command Params"(string[][] [] ("Command Params")) -> ()
  n345 = global write "WPI_DashboardLogging Global.vi" "Recording"(w41) -> ()
  n346 = local write "Command Selection"(u16 0 ("milliseconds to wait")) -> ()
  n347 = local write "Rec Mode"(w41) -> ()
